vi "Array(DBL)ToFile.vi"(0 "path":path=path "C:/misc/LabVIEW/FILES/PARAMS/OUT/by_trial01~000.psv", 2 "Array Type (2D)":enum16{"2D", "row", "column"}(ring), 3 "data format (DBL)":string="%.8f", 4 "Array(1D)":dbl[](array[numeric]) format="%_8f", 5 "Array(2D)":dbl[][](array[numeric])=[[-9.6939417702583], [-9.787461452991378], [-9.795880424049155], [-9.791754680172033], [-9.795466938501924], [-9.792349266631804], [-9.799776783437428], [-9.786104428615676], [-9.795907459503352], [-9.795268706938119], [-9.789698172547547], [-9.794336448453244], [-9.800008814538856], [-9.795556283704723], [-9.79501577752053], [-9.794266275161212], [-9.794349322608694], [-9.788410913635246], [-9.795723007815635], [-9.802258680652661], [-9.802432856674923], [-9.798080755131593], [-9.78834097315508], [-9.7946552477736], [-9.799128361260347], [-5.0269669804907995], [-9.793598741934135], [-9.784613485603533], [-9.78646503211266], [-9.792353819871323], [-9.803918973327148], [-9.80248199928148], [-9.800975798298028], [-9.785919285886518], [-9.787967678198404], [-9.792189683909982], [-9.803416273020147], [-9.785399189075022], [-9.792344159342278], [-9.799759065599373], [-9.795434869135798], [-9.798104867799251], [-9.79098036886028], [-9.80181961852864], [-9.79247681843316], [-9.778943227920282], [-9.804318999722339], [-9.786169938427546], [-9.7917473961263], [-9.787472191742584], [-9.793264780681755], [-9.796822458370732], [-9.789871238562121], [-9.799613902468865], [-9.794489448255803], [0.053253287043484795], [-9.784803341418362], [-9.795027557753857], [-9.788939930062503], [-9.79758559829949], [-9.798039859067053], [-9.80192835313501], [-9.791961705041455], [-9.796892314417502], [-9.785892415386455], [-9.797135901569282], [-9.781318785731925], [-9.796595812788555], [-9.802023321961775], [-9.799158831982991], [-9.787294065481879], [-9.79712631429669], [-9.791608695796691], [-4.671542944905596], [-9.79261449202089], [-9.80180477179711], [-9.786181349062877], [-9.792118485010652], [-9.797477226045931], [-9.78955617652576], [-9.793088478557278], [-9.797484028737504], [-9.787503430892013], [-9.789925704374266], [-9.799513676082261], [-9.787678112179325], [-9.793571042223654], [-9.80880382890866], [-9.79650163017262], [-9.79252806896738], [-0.19883449486869695], [-9.79305207299255], [-9.785793938857388], [-9.798245019409398], [-9.807212051036144], [-9.79690305644076], [-9.795699835304656], [-9.785360495953634], [-9.786913136541566], [-9.802458269440217]] format="%_8f", 6 "delimiter (\"|\")":string="|", 7 "Filename Collision Handling":T1(ring)) -> (14 "Saved":bool, 15 "File content":string="25\r\n55\r\n73\r\n90\r\n25\r\n55\r\n73\r\n90\r\n25\r\n55\r\n73\r\n90\r\n25\r\n55\r\n73\r\n90\r\n25\r\n55\r\n73\r\n90\r\n25\r\n55\r\n73\r\n90\r\n25\r\n55\r\n73\r\n90\r\n25\r\n55\r\n73\r\n90\r\n25\r\n55\r\n73\r\n90\r\n25\r\n55\r\n73\r\n90\r\n25\r\n55\r\n73\r\n90\r\n25\r\n55\r\n73\r\n90\r\n25\r\n55\r\n73\r\n90\r\n25\r\n55\r\n73\r\n90\r\n25\r\n55\r\n73\r\n90\r\n25\r\n55\r\n73\r\n90\r\n25\r\n55\r\n73\r\n90\r\n25\r\n55\r\n73\r\n90\r\n25\r\n55\r\n73\r\n90\r\n25\r\n55\r\n73\r\n90\r\n25\r\n55\r\n73\r\n90\r\n25\r\n55\r\n73\r\n90\r\n25\r\n55\r\n73\r\n90\r\n25\r\n55\r\n73\r\n90\r\n25\r\n55\r\n73\r\n90\r\n25\r\n55\r\n73\r\n90\r\n25\r\n55\r\n73\r\n90\r\n25\r\n55\r\n73\r\n90\r\n25\r\n55\r\n73\r\n90\r\n25\r\n55\r\n73\r\n90\r\n25\r\n55\r\n73\r\n90\r\n25\r\n55\r\n73\r\n90\r\n25\r\n55\r\n73\r\n90\r\n25\r\n55\r\n73\r\n90\r\n25\r\n55\r\n73\r\n90\r\n25\r\n55\r\n73\r\n90\r\n25\r\n55\r\n73\r\n90\r\n25\r\n55\r\n...")   [LabVIEW 2014]
panel:
  out "size (in bytes)":i64=4000
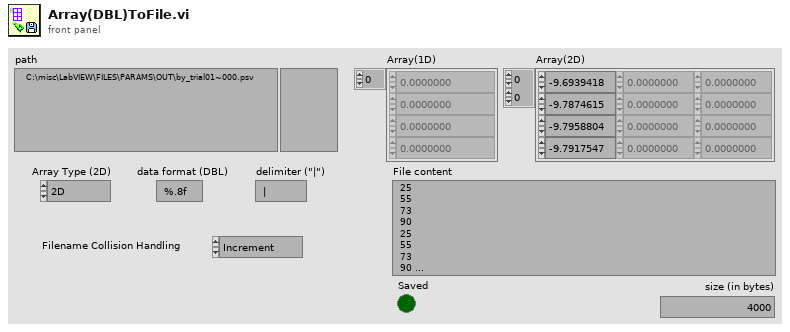
[diagram p1: front panel]
types:
  T1 = enum16{"Increment", "Overwrite", "Treat as Error"}
  T2 = enum16{"open", "replace", "create", "open or create", "replace or create", "replace or create with confirmation"}
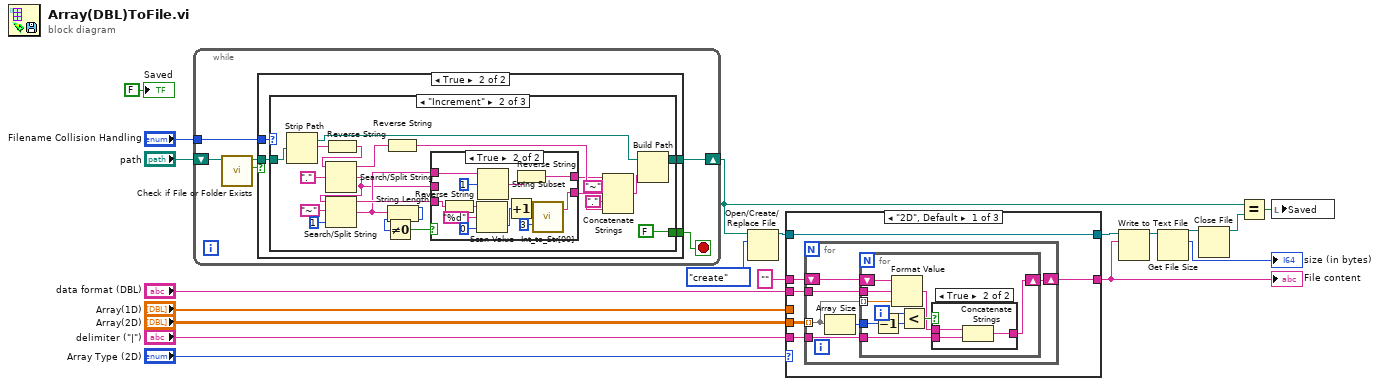
[diagram p0: block diagram]
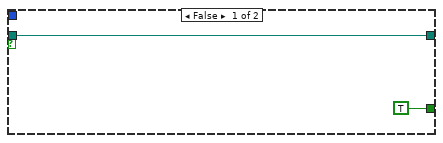
[diagram p2: hidden frame]
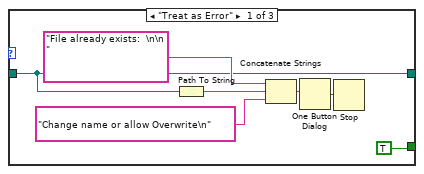
[diagram p3: hidden frame]
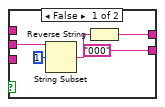
[diagram p4: hidden frame]
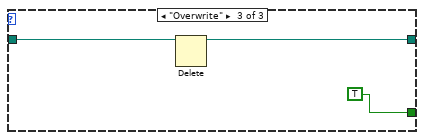
[diagram p5: hidden frame]
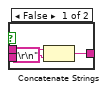
[diagram p6: hidden frame]
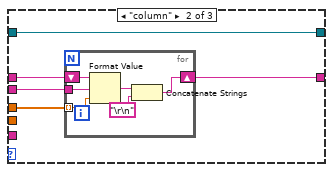
[diagram p7: hidden frame]
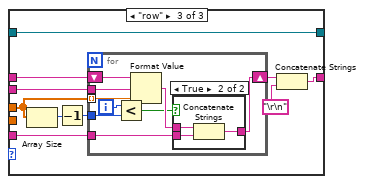
[diagram p8: hidden frame]
diagram:
  n1 = while {
    tunnel: "Filename Collision Handling" -> [w21]
    shift-right: [w22] -> w4
    shift-left: "path" -> [w25]
    stop <- w20 stop-if-true
    n2 = call <vilib>:"Check if File or Folder Exists.vi"("path"=w25) -> ("file or folder exists?"=w24:bool, "dup path"=w23:path)  [unwired: 8 in, 1 out]
    n3 = case shown="True" w24 {
      tunnel: w23 -> [w27 w31]
      tunnel: [w27 w30] -> w22
      tunnel: w21 -> [_ w29]
      tunnel: [TRUE w28] -> w20
      frame False {
      }
      frame True {
        n4 = case shown="\"Increment\"" w29 {
          tunnel: w31 -> [w35 w59 w79]
          tunnel: [w35 w43 w78] -> w30
          tunnel: [TRUE FALSE TRUE] -> w28
          frame "Treat as Error" {
            n5 = Path To String(path=w35) -> (string=w34:string)
            n6 = Concatenate Strings("File already exists:  \n\n      " ("message"), w34, "Change name or allow Overwrite\n" ("string")) -> (w37:string)
            n7 = One Button Dialog(message=w37) -> (true=w38:bool)  [unwired: 1 in]
            n8 = Stop(stop? (T)=w38) -> ()
          }
          frame "Increment" {
            n9 = Strip Path(path=w59) -> (stripped path=w44:path, name=w58:string)
            n10 = Reverse String(1:w58) -> (0:w57:string)
            n11 = Search/Split String(string=w57, search string/char (-)=".") -> (substring before match=w49:string, match + rest of string=w40:string)  [unwired: 1 in, 1 out]
            n12 = Search/Split String(string=w40, search string/char (-)="~", offset (0)=1) -> (substring before match=w52:string, match + rest of string=w41:string)  [unwired: 1 out]
            n13 = Reverse String(1:w49) -> (0:w47:string)
            n14 = String Length(string=w41) -> (length=w51:i32)
            n15 = Not Equal To 0?(x=w51) -> (x != 0?=w53:bool)
            n16 = case shown="True" w53 {
              tunnel: ["000" w71] -> w50
              tunnel: w52 -> [_ w76]
              tunnel: w41 -> [_ w66]
              tunnel: [w63 w65] -> w42
              tunnel: w40 -> [w61 _]
              frame False {
                n17 = String Subset(string=w61, offset (0)=1) -> (substring=w60:string)  [unwired: 1 in]
                n18 = Reverse String(1:w60) -> (0:w63:string)
              }
              frame True {
                n19 = Reverse String(1:w76) -> (0:w75:string)
                n20 = Scan Value(string=w75, format string="%d", default (0 dbl)=u16 0) -> (value=w72:u16)  [unwired: 1 out]
                n21 = String Subset(string=w66, offset (0)=1) -> (substring=w67:string)  [unwired: 1 in]
                n22 = Increment(x=w72) -> (x+1=w70:u16)
                n23 = Reverse String(1:w67) -> (0:w65:string)
                n24 = call "Int_to_Str[00].vi"("Positive Integer"=w70, "width (-)"=i16 3) -> ("formatted string"=w71:string)  [unwired: 17 in]
              }
            }
            n25 = Concatenate Strings(w42, "~" ("string"), w50, "." ("string"), w47) -> (w45:string)
            n26 = Build Path(base path=w44, name or relative path=w45) -> (appended path=w43:path)
          }
          frame "Overwrite" {
            n27 = Delete(path (use dialog)=w79) -> (deleted path=w78:path)  [unwired: 4 in, 2 out]
          }
        }
      }
    }
  }
  n28 = Open/Create/Replace File(file path (use dialog)=w4, operation (0:open)=T2."create") -> (refnum out=w7:refnum<file>)  [unwired: 1 in, 5 out]
  n29 = case shown="\"2D\", Default" "Array Type (2D)" {
    tunnel: "Array(1D)" -> [_ w112 w122]
    tunnel: "" -> [w84 w111 w126]
    tunnel: "delimiter (\"|\")" -> [w83 _ w125]
    tunnel: [w82 w110 w124] -> w19
    tunnel: "Array(2D)" -> [w85 _ _]
    tunnel: w7 -> [w81 w109 w123]
    tunnel: [w81 w109 w123] -> w11
    tunnel: "data format (DBL)" -> [w80 w108 w119]
    frame "2D", Default {
      n30 = for {
        tunnel: w85 -> [w90] mode=indexing
        shift-right: [w88] -> w82
        shift-left: w84 -> [w91]
        tunnel: w83 -> [w87]
        tunnel: w80 -> [w86]
        n31 = Array Size(array=w90) -> (size(s)=w89:i32)
        n32 = for {
          tunnel: w90 -> [w101] mode=indexing
          shift-right: [w94] -> w88
          shift-left: w91 -> [w100]
          tunnel: w89 -> [w97]
          tunnel: w87 -> [w93]
          tunnel: w86 -> [w92]
          i -> [w96]
          n33 = Decrement(x=w97) -> (x-1=w98:i32)
          n34 = Format Value(string ("")=w100, format string=w92, value (0)=w101) -> (output string=w95:string)
          n35 = Less?(x=w96, y=w98) -> (x < y?=w99:bool)
          n36 = case shown="True" w99 {
            tunnel: [w104 w107] -> w94
            tunnel: w95 -> [w103 w106]
            tunnel: w93 -> [_ w105]
            frame False {
              n37 = Concatenate Strings(w103, "\r\n") -> (w104:string)
            }
            frame True {
              n38 = Concatenate Strings(w106, w105) -> (w107:string)
            }
          }
        }
      }
    }
    frame "column" {
      n39 = for {
        shift-right: [w115] -> w110
        shift-left: w111 -> [w118]
        tunnel: w112 -> [w117] mode=indexing
        tunnel: w108 -> [w113]
        n40 = Format Value(string ("")=w118, format string=w113, value (0)=w117) -> (output string=w116:string)
        n41 = Concatenate Strings(w116, "\r\n") -> (w115:string)
      }
    }
    frame "row" {
      n42 = Array Size(array=w122) -> (size(s)=w121:i32)
      n43 = Decrement(x=w121) -> (x-1=w120:i32)
      n44 = for {
        shift-right: [w133] -> w127
        shift-left: w126 -> [w137]
        tunnel: w122 -> [w136] mode=indexing
        tunnel: w125 -> [w134]
        tunnel: w120 -> [w131]
        tunnel: w119 -> [w129]
        i -> [w132]
        n45 = Less?(x=w132, y=w131) -> (x < y?=w130:bool)
        n46 = Format Value(string ("")=w137, format string=w129, value (0)=w136) -> (output string=w135:string)
        n47 = case shown="True" w130 {
          tunnel: w135 -> [w138 w141]
          tunnel: w134 -> [_ w140]
          tunnel: [w138 w139] -> w133
          frame False {
          }
          frame True {
            n48 = Concatenate Strings(w141, w140) -> (w139:string)
          }
        }
      }
      n49 = Concatenate Strings(w127, "\r\n") -> (w124:string)
    }
  }
  "File content" <- w19
  n50 = Write to Text File(file (use dialog)=w11, text=w19) -> (refnum out=w10:refnum<file>)  [unwired: 2 in, 2 out]
  n51 = Get File Size(file=w10) -> (refnum out=w8:refnum<file>, size (in bytes)=→"size (in bytes)":i64)  [unwired: 1 in, 1 out]
  n52 = Close File(refnum=w8) -> (path=w5:path)  [unwired: 1 in, 1 out]
  n53 = Equal?(x=w4, y=w5) -> (x = y?=w3:bool)
  n54 = local write "Saved"(w3) -> ()
  "Saved" <- FALSE
